vi "Lift PID Raw Control.vi"(0 "Lift Potentionmeter":T6, 1 "Autonomous?":bool, 2 "Setpoint":dbl, 3 "Limit":dbl=0.666, 5 "Limit Switches":T5, 7 "Operator Gamepad":T9, 9 "Time to Wait":i32=10, 11 "From Shift":dbl, 12 "Gains UP":cluster{"P":dbl, "I":dbl, "D":dbl}={"P"=0.1, "I"=0.0, "D"=0.0}, 13 "Gains DOWN":cluster{"P":dbl, "I":dbl, "D":dbl}={"P"=0.1, "I"=0.0, "D"=0.0}, 14 "Lift Deadband":dbl=0.1) -> (4 "Lift Potentiometer Out":T6, 6 "Limit Switches Out":T5, 8 "Motor output":dbl format="%#_13g", 10 "Tolerable?":bool, 15 "To Shift":dbl)   [LabVIEW 2014]
uses:
  <vilib>/Rock Robotics/WPI/Joystick/WPI_JoystickDevRef.ctl
  <vilib>/Rock Robotics/WPI/Joystick/WPI_JoystickDeviceEnum.ctl
  <vilib>/Rock Robotics/WPI/Potentiometer/WPI_PotentiometerDevRef.ctl
  <vilib>/Rock Robotics/SystemInterfaces/Typedef/FPGA_TypedefAnalogModule.ctl
  <vilib>/Rock Robotics/SystemInterfaces/AI/FPGA_AIChannel.ctl
  <vilib>/Rock Robotics/WPI/Switch/WPI_SwitchDevRef.ctl
  <vilib>/Rock Robotics/SystemInterfaces/DIO/FPGA_DIOChannel.ctl
  <vilib>/Rock Robotics/SystemInterfaces/Typedef/FPGA_TypedefDigitalModule.ctl
  <vilib>/Rock Robotics/SystemInterfaces/Counter/FPGA_CounterCtrSystemIndex.ctl
  <vilib>/Rock Robotics/WPI/DriverStation/WPI_DriverStationRobotMode2.ctl
  Robot Global Data.vi
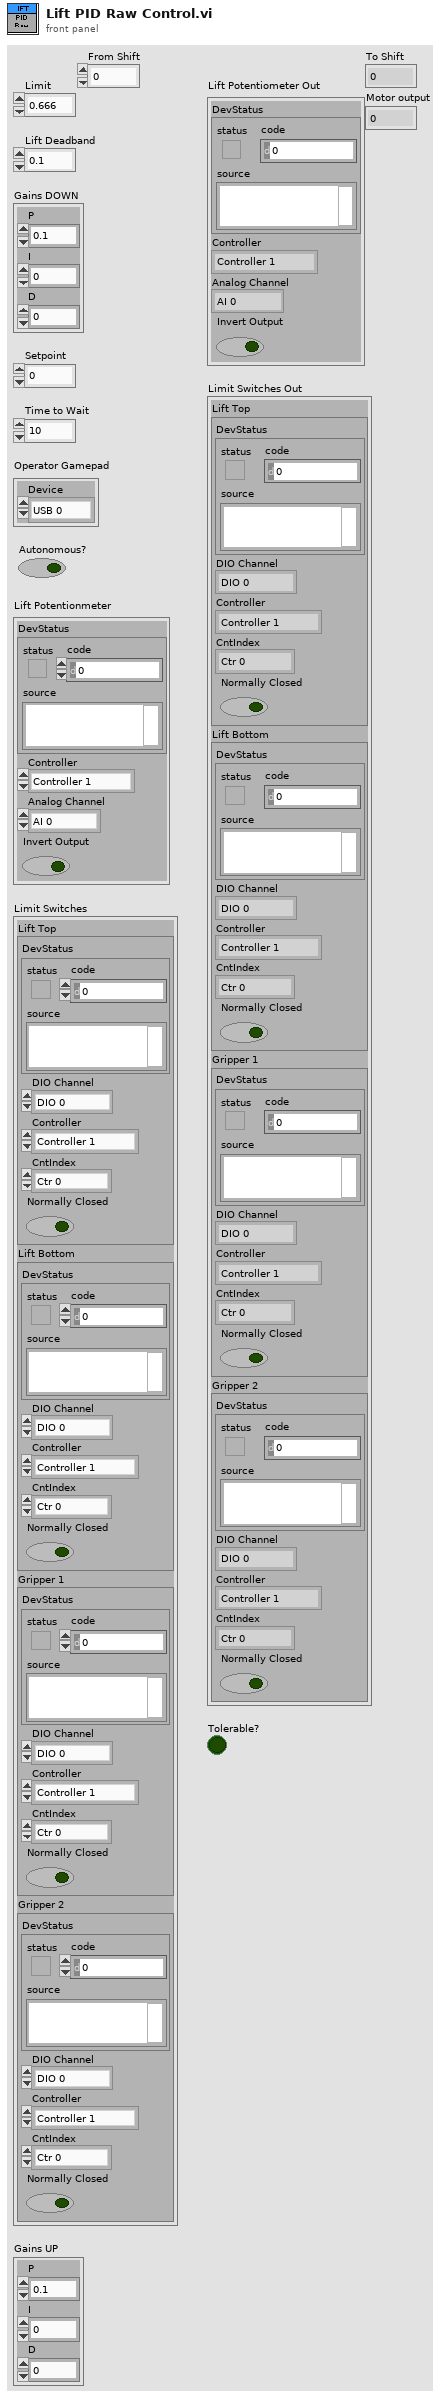
[diagram p1: front panel]
types:
  T1 = typedef "WPI_SwitchDevRef.ctl" = cluster{"DevStatus":errorcluster, "DIO Channel":T2, "Controller":T3, "CntIndex":T4, "Normally Closed":bool}
  T2 = typedef "FPGA_DIOChannel.ctl" = enum8{"DIO 0", "DIO 1", "DIO 2", "DIO 3", "DIO 4", "DIO 5", "DIO 6", "DIO 7", "DIO 8", "DIO 9", "DIO MXP 0", "DIO MXP 1", "DIO MXP 2", "DIO MXP 3", "DIO MXP 4", "DIO MXP 5", "DIO MXP 6", "DIO MXP 7", "DIO MXP 8", "DIO MXP 9", "DIO MXP 10", "DIO MXP 11", "DIO MXP 12", "DIO MXP 13", "DIO MXP 14", "DIO MXP 15", "Invalid"}
  T3 = typedef "FPGA_TypedefDigitalModule.ctl" = enum16{"Controller 1"}
  T4 = typedef "FPGA_CounterCtrSystemIndex.ctl" = enum8{"Ctr 0", "Ctr 1", "Ctr 2", "Ctr 3", "Ctr 4", "Ctr 5", "Ctr 6", "Ctr 7", "Invalid"}
  T5 = cluster{"Lift Top":T1, "Lift Bottom":T1, "Gripper 1":T1, "Gripper 2":T1}
  T6 = typedef "WPI_PotentiometerDevRef.ctl" = cluster{"DevStatus":errorcluster, "Controller":T7, "Analog Channel":T8, "Invert Output":bool}
  T7 = typedef "FPGA_TypedefAnalogModule.ctl" = enum16{"Controller 1"}
  T8 = typedef "FPGA_AIChannel.ctl" = enum8{"AI 0", "AI 1", "AI 2", "AI 3", "AI MXP 0", "AI MXP 1", "AI MXP 2", "AI MXP 3", "Invalid"}
  T9 = typedef "WPI_JoystickDevRef.ctl" = cluster{"Device":T10}
  T10 = typedef "WPI_JoystickDeviceEnum.ctl" = enum16{"USB 0", "USB 1", "USB 2", "USB 3", "USB 4", "USB 5"}
  T11 = typedef "WPI_DriverStationRobotMode2.ctl" = enum16{"Autonomous Disabled", "Autonomous Enabled", "Teleop Disabled", "Teleop Enabled", "Disconnected", "Finish", "Test Disabled", "Test Enabled", "Emergency Stopped"}
  T12 = cluster{"Error":dbl, "millisecond timer value":u32, "To Shift Register":dbl}
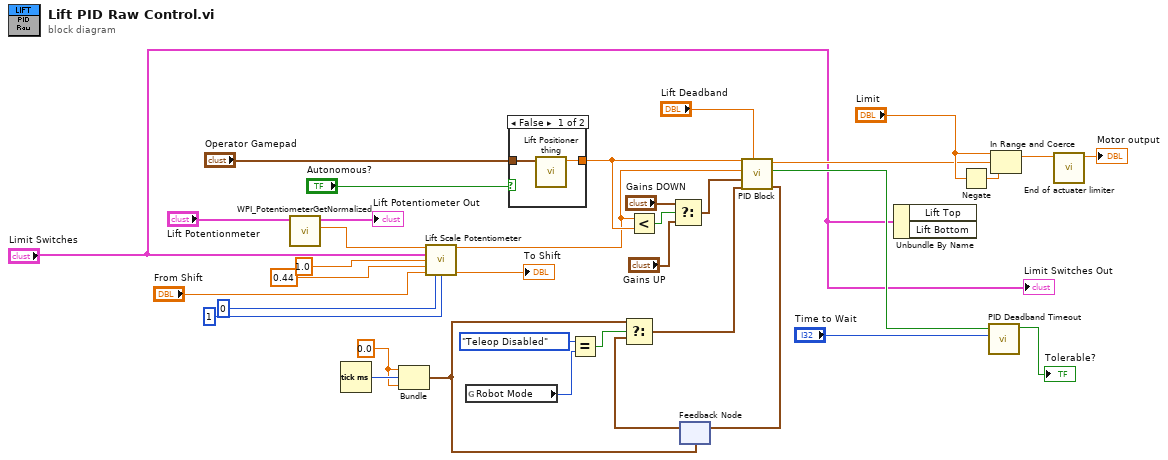
[diagram p0: block diagram]
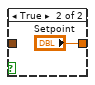
[diagram p2: hidden frame]
diagram:
  w20 = 0.0
  n1 = call <vilib>:"WPI_PotentiometerGetNormalized.vi"("PotDevRef"="Lift Potentionmeter") -> ("Normalized Value"=w10:dbl, "PotDevRef"=→"Lift Potentiometer Out":T6)  [unwired: 8 in, 1 out]
  n2 = Tick Count (ms)() -> (millisecond timer value=w21:u32)
  n3 = Bundle(w20, "millisecond timer value"=w21, w20) -> (w24:cluster{dbl, "millisecond timer value":u32, dbl})  [unwired: 1 in]
  n4 = call "Lift Scale Potentiometer.vi"("Potentiometer In"=w10, "Limit Switches"="Limit Switches", "Initial Upper Value"=1.0, "Initial Lower Value"=0.44 ("y"), "From Shift"="From Shift", "Upper Limit Index ( 0 - 3 )"=0 ("Upper Limit Index ( 1 - 4 )"), "Lower Limit Index (0 - 3 )"=1 ("Upper Limit Index ( 1 - 4 )")) -> ("Scaled Value Out"=w5:dbl, "To Shift"=→"To Shift":dbl)  [unwired: 7 in]
  n5 = global read "Robot Global Data.vi" "Robot Mode"() -> (w27:T11)
  n6 = case shown="False" "Autonomous?" {
    tunnel: "Operator Gamepad" -> [w38 _]
    tunnel: [w37 "Setpoint"] -> w34
    frame False {
      n7 = call "Lift Positioner thing.vi"("Operator Gamepad"=w38) -> ("Setpoint"=w37:dbl)  [unwired: 10 in]
    }
    frame True {
    }
  }
  n8 = Equal?(x=WPI_DriverStationRobotMode2."Teleop Disabled", y=w27) -> (x = y?=w25:bool)
  n9 = Less?(x=w5, y=w34) -> (x < y?=w32:bool)
  n10 = Select(t="Gains DOWN", s=w32, f="Gains UP") -> (s? t:f=w33:cluster{"P":dbl, "I":dbl, "D":dbl})
  n11 = feedback #1(w24) -> (w23:cluster{dbl, "millisecond timer value":u32, dbl})
  n12 = Select(t=w24, s=w25, f=w23) -> (s? t:f=w22:cluster{dbl, "millisecond timer value":u32, dbl})
  n13 = call "PID Block.vi"("Deadband"="Lift Deadband", "From Shift"=w22, "Gains"=w33, "Position"=w5, "Setpoint"=w34) -> ("To Shift"=w12:T12, "Tolerable?"=w13:bool, "Output"=w16:dbl)  [unwired: 4 in]
  n14 = feedback-in #1(w12) -> ()
  n15 = Unbundle By Name("Limit Switches") -> ()  [unwired: 2 out]
  n16 = Negate(x="Limit") -> (-x=w18:dbl)
  n17 = call "PID Deadband Timeout.vi"("Time to Wait"="Time to Wait", "In deadband range?"=w13) -> ("Deadband Timed-out"=→"Tolerable?":bool)  [unwired: 9 in]
  n18 = In Range and Coerce(upper limit="Limit", x=w16, lower limit=w18) -> (coerced(x)=w17:dbl)  [unwired: 1 out]
  n19 = call "End of actuater limiter.vi"("Motor input"=w17) -> ("Motor output"=→"Motor output":dbl)  [unwired: 10 in]
  "Limit Switches Out" <- "Limit Switches"
